vi "Create All Message Queues.vi"(8 "error in (no error)":errorcluster) -> (0 "error out":errorcluster, 3 "Message Queues out":T1)   [LabVIEW 2019, in "Message Named Queue.lvlib"]
doc: "This VI creates and initializes all the message queues for your application. If your application requires more than one message queue, right-click the \"Message Queues\" constant above and select Open Type Def. Add the new Message Queue(s) to the type definition, then initialize them in this VI."
uses:
  Message Named Queue.lvlib
  All Message Queues.ctl
  Message Cluster.ctl
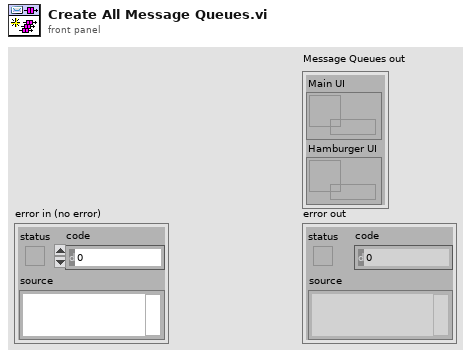
[diagram p1: front panel]
types:
  T1 = typedef "Message Named Queue.lvlib/All Message Queues.ctl" = cluster{"Main UI":refnum<queue>, "Hamburger UI":refnum<queue>}
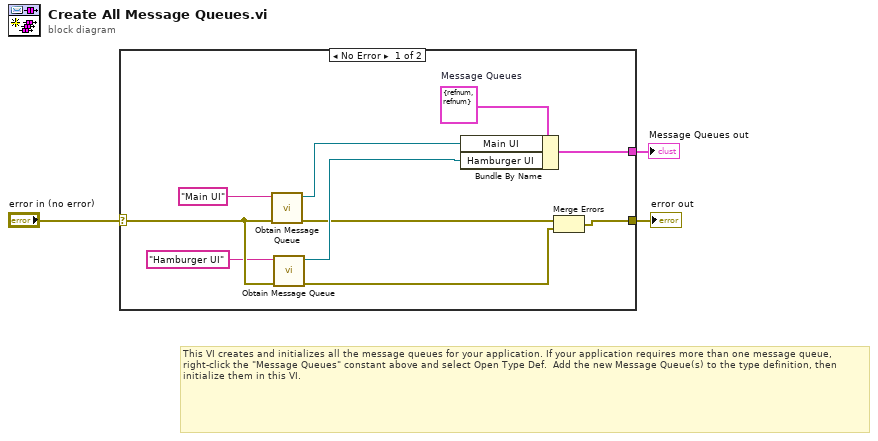
[diagram p0: block diagram]
diagram:
  # "This VI creates and initializes all the message queues for your application. If your application requires more than one message queue, right-click the \"Message Queues\" constant above and select Open Type Def.  Add the new Message Queue(s) to the type definition, then initialize them in this VI."
  n1 = case shown="No Error" "error in (no error)" {
    selector: "error in (no error)" -> [w9 w14]
    tunnel: [w8 w14] -> w3
    tunnel: [w12 _] -> w2
    frame No Error {
      w13 = T1 {"Main UI"=refnum, "Hamburger UI"=refnum}  # Message Queues
      n2 = call "Obtain Message Queue.vi"("error in (no error)"=w9, "Queue name"="Main UI") -> ("error out"=w4:errorcluster, "Message Queue"=w11:refnum<queue>)  [unwired: 8 in]
      n3 = call "Obtain Message Queue.vi"("error in (no error)"=w9, "Queue name"="Hamburger UI") -> ("error out"=w7:errorcluster, "Message Queue"=w10:refnum<queue>)  [unwired: 8 in]
      n4 = Bundle By Name(cluster=w13, "Main UI"=w11, "Hamburger UI"=w10) -> (w12:T1)
      n5 = Merge Errors(w4, w7) -> (w8:errorcluster)
    }
    frame Error {
    }
  }
  "Message Queues out" <- w2
  "error out" <- w3
